vi "getApproxVector.vi"(10 "xi":dbl[](array[numeric]), 11 "data wire":T1 {"x locations" format="%.4g"; "coefficients" format="%.4g"}) -> (2 "yi":dbl[](array[numeric]))   [LabVIEW 2014]
uses:
  <vilib>/gmath/interp.llb/in_piecewise interp poly control.ctl
  <vilib>/gmath/NI_Gmath.lvlib
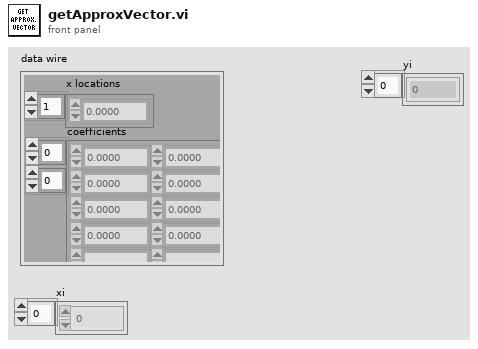
[diagram p1: front panel]
types:
  T1 = typedef "NI_Gmath.lvlib/in_piecewise interp poly control.ctl" = cluster{"x locations":dbl[], "coefficients":dbl[][]}
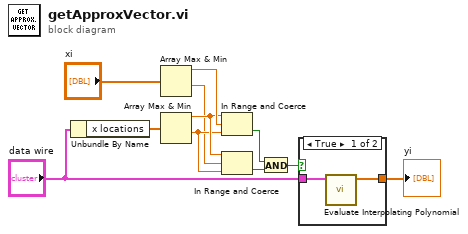
[diagram p0: block diagram]
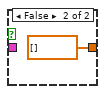
[diagram p2: hidden frame]
diagram:
  n1 = Unbundle By Name("data wire") -> ("x locations"=w11:dbl[])
  n2 = Array Max & Min(array="xi") -> (max value=w8:dbl, min value=w5:dbl)  [unwired: 2 out]
  n3 = Array Max & Min(array=w11) -> (max value=w7:dbl, min value=w6:dbl)  [unwired: 2 out]
  n4 = In Range and Coerce(upper limit=w7, x=w8, lower limit=w6) -> (In Range?=w4:bool)  [unwired: 1 out]
  n5 = In Range and Coerce(upper limit=w7, x=w5, lower limit=w6) -> (In Range?=w3:bool)  [unwired: 1 out]
  n6 = And(x=w4, y=w3) -> (x .and. y?=w2:bool)
  n7 = case shown="True" w2 {
    tunnel: "data wire" -> [w13 _]
    tunnel: [w12 dbl[] [] ("yi")] -> w1
    frame True {
      n8 = call <vilib>:"Evaluate Interpolating Polynomial.vi"("piecewise polynomial"=w13) -> ("yi"=w12:dbl[])  [unwired: 9 in, 1 out]
    }
    frame False {
    }
  }
  "yi" <- w1
